vi "MultiChannel Write.vi"(8 "Error In":errorcluster, 10 "Data to Log":dbl[][](array[numeric]), 11 "File Refnum In":refnum<file>) -> (0 "Error Out":errorcluster, 3 "File Refnum Out":refnum<file>)   [LabVIEW 2012]
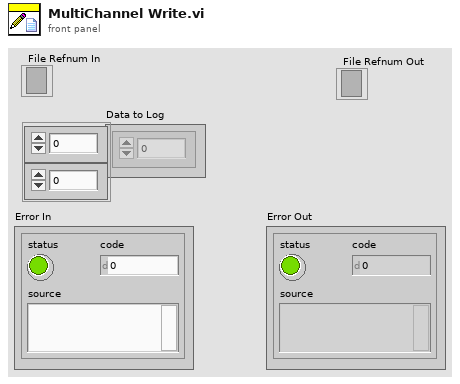
[diagram p1: front panel]
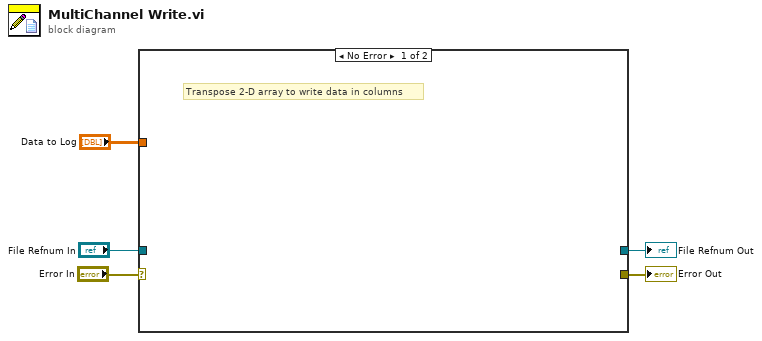
[diagram p0: block diagram]
diagram:
  n1 = case shown="No Error" "Error In" {
    selector: "Error In" -> [_ w7]
    tunnel: "File Refnum In" -> [_ w6]
    tunnel: [_ w6] -> w3
    tunnel: [_ w7] -> w2
    tunnel: "Data to Log" -> [_ _]
    frame No Error {
      # "Transpose 2-D array to write data in columns"
    }
    frame Error {
    }
  }
  "Error Out" <- w2
  "File Refnum Out" <- w3
